vi "Write_parameter.vi"(8 "error in (no error)":errorcluster caption="entrée d'erreur (pas d'erreur)", 10 "Parameter":string, 11 "Class Relay_Board en entrée":refnum<class "Class Instrument UART.lvclass">) -> (0 "error out":errorcluster caption="sortie d'erreur", 3 "Class Relay_Board en Sortie":refnum<class "Class Instrument UART.lvclass">)   [LabVIEW 2020, in "Library Instrument & Equipement.lvlib" / "Library Instruments.lvlib" / "Class Instrument UART.lvclass"]
uses:
  Class Instrument UART.lvclass
  Commun VI/TypeDef/Commande UART/Parametre UART.ctl
  UART/UART (Default)/Class UART (Default).lvclass
  JSON API/JSON Value/Set from JSON string.vi
  Instrument (Default)/Class Instrument (Default).lvclass
  JSON API/JSON Value/JSON Value.lvclass
  Class Instrument UART.lvclass/Class Instrument UART.ctl
  JSON API/Variant JSON/Variant JSON.lvlib
  JSON API/Get Polymorphic/JSON GetSet.lvlib
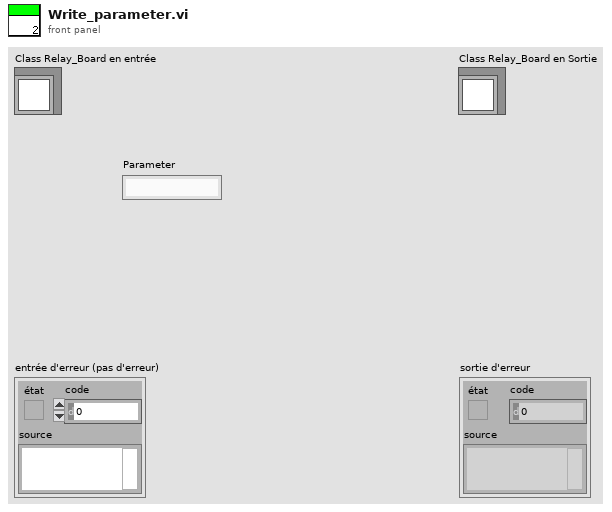
[diagram p1: front panel]
types:
  T1 = typedef "Parametre UART.ctl" = cluster{"Address Device":refnum<visa-resource-name>, "Baud Rate":u32, "Data Bit":u16, "stop bits (10: 1 bit)":u16, "parity (0:none)":enum16{"None", "Odd", "Even", "Mark", "Space"}, "flow control (0:none)":u16, "termination char ":u8, "Enable Termination":bool, "Nb Octet to Read":u16, "Class UART":refnum<class "Class UART (Default).lvclass">}
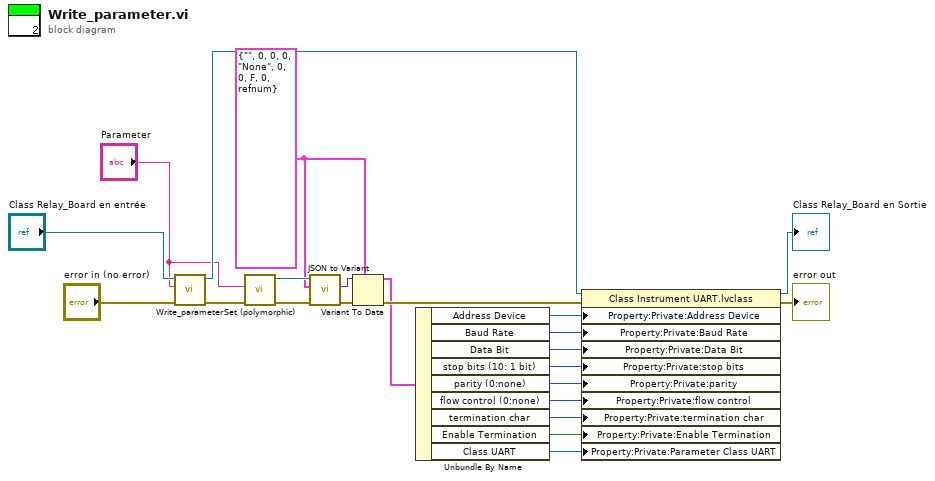
[diagram p0: block diagram]
diagram:
  w10 = T1 {"Address Device"="", "Baud Rate"=0, "Data Bit"=0, "stop bits (10: 1 bit)"=0, "parity (0:none)"=enum."None", "flow control (0:none)"=0, "termination char "=0, "Enable Termination"=FALSE, "Nb Octet to Read"=0, "Class UART"=refnum} ("Parameter")
  n1 = call-parent "Write_parameter.vi"("error in (no error)"="error in (no error)", "Parameter"="Parameter", "Class Instrument (Default) en entrée"="Class Relay_Board en entrée") -> ("error out"=w14:errorcluster, "Class Instrument (Default) en sortie"=w12:refnum<class "Class Instrument UART.lvclass">)  [unwired: 7 in]
  n2 = call-poly "Set (polymorphic).vi"("error in (no error)"=w14, "JSON stream"="Parameter") -> ("error out"=w21:errorcluster, "JSON Value out"=w23:refnum<class "JSON Value.lvclass">)  [unwired: 7 in, 1 out]
  n3 = call "JSON to Variant.vi"("error in (no error)"=w21, "Variant (Data Type)"=w10, "JSON Value"=w23) -> ("error out"=w22:errorcluster, "Variant out"=w20:variant)  [unwired: 7 in]
  n4 = Variant To Data(error in=w22, type=w10, Variant=w20) -> (data=w15:T1, error out=w16:errorcluster)
  n5 = Unbundle By Name(w15) -> ("Address Device"=w9:refnum<visa-resource-name>, "Baud Rate"=w8:u32, "Data Bit"=w7:u16, "stop bits (10: 1 bit)"=w6:u16, "parity (0:none)"=w5:enum16{"None", "Odd", "Even", "Mark", "Space"}, "flow control (0:none)"=w4:u16, "termination char"=w3:u8, "Enable Termination"=w2:bool, "Class UART"=w1:refnum<class "Class UART (Default).lvclass">)
  n6 = property class="Class Instrument UART.lvclass"(reference=w12, error in=w16, "Property:Private:Address Device"=w9, "Property:Private:Baud Rate"=w8, "Property:Private:Data Bit"=w7, "Property:Private:stop bits"=w6, "Property:Private:parity"=w5, "Property:Private:flow control"=w4, "Property:Private:termination char "=w3, "Property:Private:Enable Termination"=w2, "Property:Private:Parameter Class UART"=w1) -> (reference out=→"Class Relay_Board en Sortie":refnum<class "Class Instrument UART.lvclass">, error out=→"error out":errorcluster)
